vi "Update Limits File.vi"(0 "Session Handle in":T4, 7 "Evaluations In":T1[](array[typedef]) {"Low Limit" format="%#_13g"; "SI Scaling" items=["femto"=-15, "pico"=-12, "nano"=-9, "micro"=-6, "milli"=-3, "percent"=-2, ""=0, "kilo"=3, "mega"=6, "giga"=9, "tera"=12]}, 11 "error in (no error)":errorcluster) -> (4 "Session Handle out":T4, 15 "error out":errorcluster)   [LabVIEW 2018, in "Test Number and Bin Generator.lvlib" / "Test Number and Bin Generator.lvclass"]
uses:
  Test Number and Bin Generator.lvclass
  Typedefs/Session Handle.ctl
  Plugins/TestStand API Tools (TSAT).lvlibp/Evaluation Actions/Includes/Controls/TSAT Evaluation.ctl
  Plugins/TestStand API Tools (TSAT).lvlibp/Evaluation Actions/Includes/Controls/TSAT Eval SI Unit Scaling.ctl
  Plugins/TestStand API Tools (TSAT).lvlibp/Evaluation Actions/Includes/Controls/TSAT Evaluation Type.ctl
  Plugins/TestStand API Tools (TSAT).lvlibp/Evaluation Actions/TSAT Evaluation Actions.lvlib
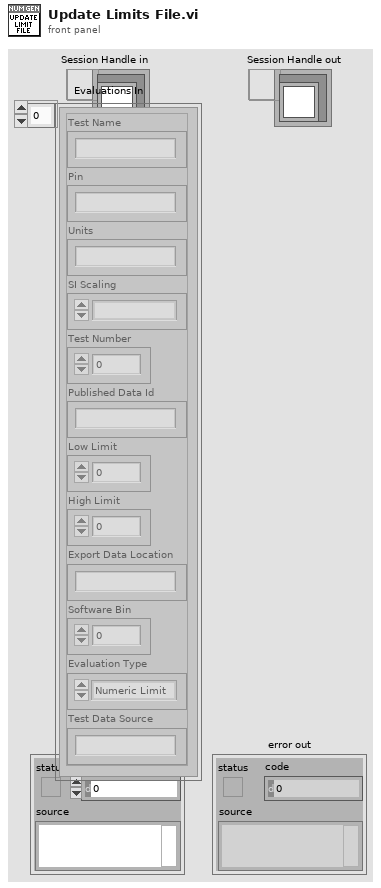
[diagram p1: front panel]
types:
  T1 = typedef "TestStand API Tools (TSAT).lvlibp/TSAT Evaluation Actions.lvlib/TSAT Evaluation.ctl" = cluster{"Test Name":string, "Pin":string, "Units":string, "SI Scaling":T2, "Test Number":i32, "Published Data Id":string, "Low Limit":dbl, "High Limit":dbl, "Export Data Location":string, "Software Bin":i64, "Evaluation Type":T3, "Test Data Source":string}
  T2 = typedef "TestStand API Tools (TSAT).lvlibp/TSAT Evaluation Actions.lvlib/TSAT Eval SI Unit Scaling.ctl" = i16
  T3 = typedef "TestStand API Tools (TSAT).lvlibp/TSAT Evaluation Actions.lvlib/TSAT Evaluation Type.ctl" = enum16{"Numeric Limit", "Pass/Fail", "None"}
  T4 = typedef "Test Number and Bin Generator.lvlib/Test Number and Bin Generator.lvclass/Session Handle.ctl" = refnum<data-value>
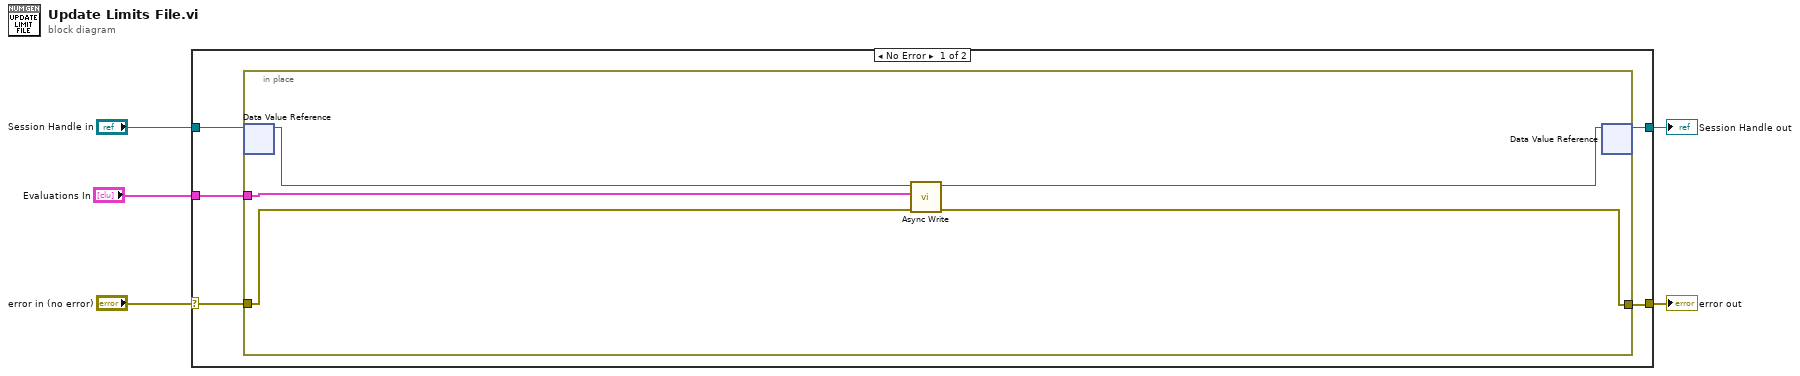
[diagram p0: block diagram]
diagram:
  n1 = case shown="No Error" "error in (no error)" {
    selector: "error in (no error)" -> [w8 w16]
    tunnel: "Session Handle in" -> [w10 w17]
    tunnel: [w9 w17] -> w4
    tunnel: [w6 w16] -> w3
    tunnel: "Evaluations In" -> [w7 _]
    frame No Error {
      n2 = in-place {
        in-place-border: w8 -> [w11]
        in-place-border: w7 -> [w15]
        in-place-border: [w14] -> w6
        n3 = in-place-dvr #1(w10) -> (w12:refnum<class "Test Number and Bin Generator.lvclass">)  [unwired: 1 out]
        n4 = call "Async Write.vi"("error in (no error)"=w11, "Evaluations In"=w15, "Test Number and Bin Generator in"=w12) -> ("error out"=w14:errorcluster, "Test Number and Bin Generator out"=w13:refnum<class "Test Number and Bin Generator.lvclass">)  [unwired: 7 in]
        n5 = in-place-dvr #1(w13) -> (w9:T4)  [unwired: 1 out]
      }
    }
    frame Error {
    }
  }
  "Session Handle out" <- w4
  "error out" <- w3
